vi "DeviceOn.vi"(8 "error in (no error)":errorcluster, 11 "PacificPowerSource in":refnum<class "PacificPowerSource.lvclass">) -> (0 "error out":errorcluster, 3 "PacificPowerSource out":refnum<class "PacificPowerSource.lvclass">)   [LabVIEW 2018, in "AcPwrPlugins.lvlib" / "PacificPowerSource.lvclass"]
doc: "This VI sets the output to on by closing the output switch."
uses:
  PacificPowerSource.lvclass
  <instrlib>/Pacific Power UPC Series/Pacific Power UPC Series.lvlib
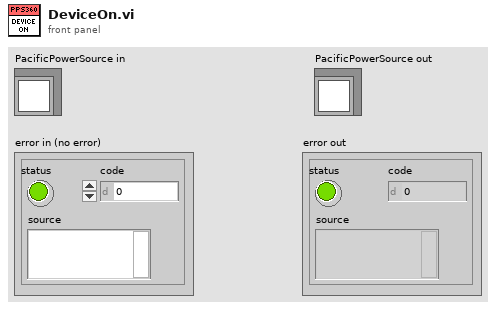
[diagram p1: front panel]
types:
  T1 = typedef "AcPwrPlugins.lvlib/PacificPowerSource.lvclass/Device(s)Settings.ctl" = cluster{"MeasName":string, "Modules":cluster{"Handle":string, "Connected":bool, "Clear Device (F)":bool, "btnIdQuery":bool, "btnReset":bool, "Program #":cluster{"Phase B (Degrees)":i32, "Waveform A (1: Sine)":i32, "Voltage Level (Va)":dbl, "Program Number (0)":i32, "Voltage Level (Vb) ":dbl, "Form (3: Three)":u16, "Coupling  (0: Direct)":u16, "Frequency (45Hz)":dbl, "Current Limit (40A)":dbl, "Phase C (Degrees)":i32, "Voltage Level (Vc)":dbl, "Waveform B (1: Sine)":i32, "Waveform C (1: Sine)":i32}[], "Impedance Parameters (off, 0.00)":cluster{"State":bool, "Impedance":dbl}, "Transient Execution (F)":bool, "OutputEnabled":bool, "Source Range":cluster{"Frequency Minimum (45 Hz)":dbl, "Frequency Maximum (1200 Hz)":dbl, "Voltage Maximum (V)":dbl, "Voltage Minimum (V)":dbl, "Range Control (0: Auto)":u16, "Initial Voltage (0V)":u16, "Frequency Range (600Hz)":u16}, "Port Type":enum16{"GPIB", "Serial"}}[]}
  T2 = typedef "AcPwrPlugins.lvlib/PacificPowerSource.lvclass/Measurements.ctl" = cluster{"Handle":string, "Name":string, "Enabled ":bool, "Measurement Value":dbl, "Channel Name":enum16{"A", "B", "C"}, "Measurement Type ":T3}[]
  T3 = typedef "AcPwrPlugins.lvlib/PacificPowerSource.lvclass/MeasurementType.ctl" = enum16{"Voltage RMS L-N", "Voltage RMS L-L", "Frequency", "Current RMS", "Current Peak", "Crest Factor", "Power Factor", "Power VA", "Real Power"}
  T4 = typedef "AcPwrPlugins.lvlib/PacificPowerSource.lvclass/Modules.ctl" = cluster{"Handle":string, "Connected":bool, "Clear Device (F)":bool, "btnIdQuery":bool, "btnReset":bool, "Program #":cluster{"Phase B (Degrees)":i32, "Waveform A (1: Sine)":i32, "Voltage Level (Va)":dbl, "Program Number (0)":i32, "Voltage Level (Vb) ":dbl, "Form (3: Three)":u16, "Coupling  (0: Direct)":u16, "Frequency (45Hz)":dbl, "Current Limit (40A)":dbl, "Phase C (Degrees)":i32, "Voltage Level (Vc)":dbl, "Waveform B (1: Sine)":i32, "Waveform C (1: Sine)":i32}[], "Impedance Parameters (off, 0.00)":cluster{"State":bool, "Impedance":dbl}, "Transient Execution (F)":bool, "OutputEnabled":bool, "Source Range":cluster{"Frequency Minimum (45 Hz)":dbl, "Frequency Maximum (1200 Hz)":dbl, "Voltage Maximum (V)":dbl, "Voltage Minimum (V)":dbl, "Range Control (0: Auto)":u16, "Initial Voltage (0V)":u16, "Frequency Range (600Hz)":u16}, "Port Type":enum16{"GPIB", "Serial"}}[]
  T5 = cluster{"Phase B (Degrees)":i32, "Waveform A (1: Sine)":i32, "Voltage Level (Va)":dbl, "Program Number (0)":i32, "Voltage Level (Vb) ":dbl, "Form (3: Three)":u16, "Coupling  (0: Direct)":u16, "Frequency (45Hz)":dbl, "Current Limit (40A)":dbl, "Phase C (Degrees)":i32, "Voltage Level (Vc)":dbl, "Waveform B (1: Sine)":i32, "Waveform C (1: Sine)":i32}[]
  T6 = cluster{"Phase B (Degrees)":i32, "Waveform A (1: Sine)":i32, "Voltage Level (Va)":dbl, "Program Number (0)":i32, "Voltage Level (Vb) ":dbl, "Form (3: Three)":u16, "Coupling  (0: Direct)":u16, "Frequency (45Hz)":dbl, "Current Limit (40A)":dbl, "Phase C (Degrees)":i32, "Voltage Level (Vc)":dbl, "Waveform B (1: Sine)":i32, "Waveform C (1: Sine)":i32}
  T7 = cluster{"Handle":string, "Connected":bool, "Clear Device (F)":bool, "btnIdQuery":bool, "btnReset":bool, "Program #":cluster{"Phase B (Degrees)":i32, "Waveform A (1: Sine)":i32, "Voltage Level (Va)":dbl, "Program Number (0)":i32, "Voltage Level (Vb) ":dbl, "Form (3: Three)":u16, "Coupling  (0: Direct)":u16, "Frequency (45Hz)":dbl, "Current Limit (40A)":dbl, "Phase C (Degrees)":i32, "Voltage Level (Vc)":dbl, "Waveform B (1: Sine)":i32, "Waveform C (1: Sine)":i32}[], "Impedance Parameters (off, 0.00)":cluster{"State":bool, "Impedance":dbl}, "Transient Execution (F)":bool, "OutputEnabled":bool, "Source Range":cluster{"Frequency Minimum (45 Hz)":dbl, "Frequency Maximum (1200 Hz)":dbl, "Voltage Maximum (V)":dbl, "Voltage Minimum (V)":dbl, "Range Control (0: Auto)":u16, "Initial Voltage (0V)":u16, "Frequency Range (600Hz)":u16}, "Port Type":enum16{"GPIB", "Serial"}}
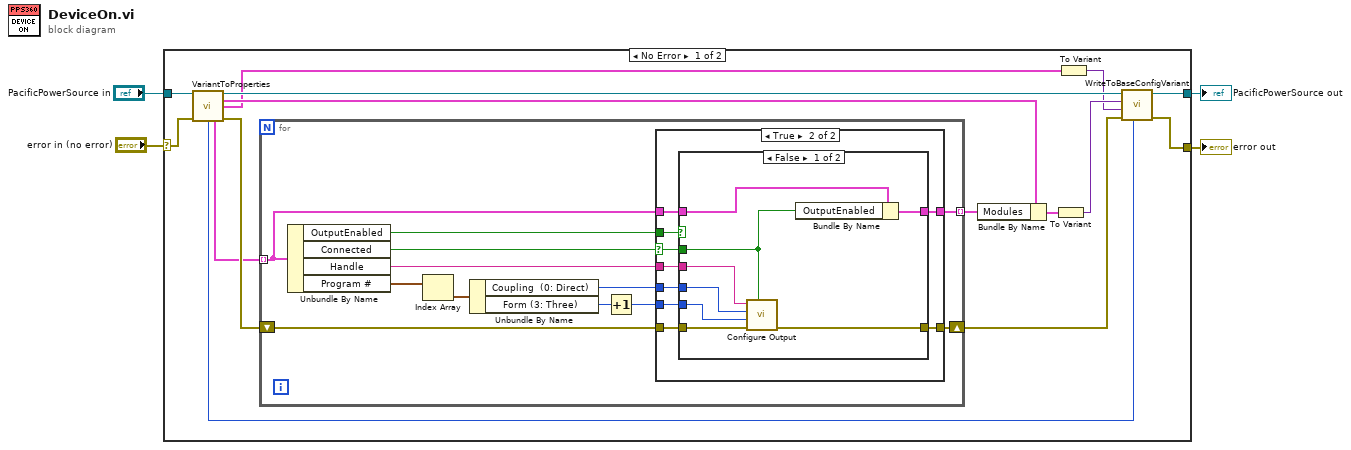
[diagram p0: block diagram]
diagram:
  n1 = case shown="No Error" "error in (no error)" {
    selector: "error in (no error)" -> [w19 w54]
    tunnel: [w9 w54] -> w1
    tunnel: [w8 w53] -> w2
    tunnel: "PacificPowerSource in" -> [w11 w53]
    frame No Error {
      n2 = call "VariantToProperties.vi"("PacificPowerSource in"=w11, "error in (no error)"=w19) -> ("PacificPowerSource out"=w10:refnum<class "PacificPowerSource.lvclass">, "Device(s)Settings"=w13:T1, "Measurements"=w5:T2, "Measurement Refresh Time (ms)"=w6:u32, "Modules"=w14:T4, "error out"=w17:errorcluster)  [unwired: 7 in, 1 out]
      n3 = for {
        tunnel: w14 -> [w27] mode=indexing
        shift-right: [w29] -> w15
        shift-left: w17 -> [w28]
        tunnel: [w26] -> w18 mode=indexing
        n4 = Unbundle By Name(w27) -> ("OutputEnabled"=w25:bool, "Connected"=w30:bool, "Handle"=w31:string, "Program #"=w24:T5)
        n5 = Index Array(array=w24) -> (element=w23:T6)  [unwired: 1 in]
        n6 = Unbundle By Name(w23) -> ("Coupling  (0: Direct)"=w22:u16, "Form (3: Three)"=w21:u16)
        n7 = Increment(x=w21) -> (x+1=w20:u16)
        n8 = case shown="True" w30 {
          selector: w30 -> [_ w38]
          tunnel: w28 -> [w33 w42]
          tunnel: [w33 w41] -> w29
          tunnel: w31 -> [_ w40]
          tunnel: w27 -> [w32 w39]
          tunnel: [w32 w37] -> w26
          tunnel: w25 -> [_ w36]
          tunnel: w22 -> [_ w35]
          tunnel: w20 -> [_ w34]
          frame False {
          }
          frame True {
            n9 = case shown="False" w36 {
              tunnel: w42 -> [w50 w51]
              tunnel: [w49 w51] -> w41
              tunnel: w40 -> [w48 _]
              tunnel: w39 -> [w43 w52]
              tunnel: w38 -> [w47 _]
              tunnel: [w46 w52] -> w37
              tunnel: w35 -> [w45 _]
              tunnel: w34 -> [w44 _]
              frame False {
                n10 = call <instrlib>:"Configure Output.vi"("Enable Output (T: Enable)"=w47, "error in (no error)"=w50, "Form (3: Three)"=w44, "Coupling  (0: Direct)"=w45, "VISA resource name"=w48) -> ("error out"=w49:errorcluster)  [unwired: 5 in, 1 out]
                n11 = Bundle By Name(cluster=w43, "OutputEnabled"=w47) -> (w46:T7)
              }
              frame True {
              }
            }
          }
        }
      }
      n12 = Bundle By Name(cluster=w13, "Modules"=w18) -> (w12:T1)
      n13 = To Variant(anything=w12) -> (Variant=w16:variant)
      n14 = To Variant(anything=w5) -> (Variant=w7:variant)
      n15 = call "WriteToBaseConfigVariant.vi"("Measurement Refresh Time (ms)"=w6, "error in (no error)"=w15, "Meas"=w7, "Config"=w16, "PacificPowerSource in"=w10) -> ("error out"=w9:errorcluster, "PacificPowerSource out"=w8:refnum<class "PacificPowerSource.lvclass">)  [unwired: 5 in]
    }
    frame Error {
    }
  }
  "error out" <- w1
  "PacificPowerSource out" <- w2
